vi "MapURLCreation.vi"(1 "Longitude":dbl=-1.307 format="%#.6g", 2 "Latitude":dbl=51.4062 format="%#.6g") -> (0 "URL":string="http://maps.google.com/staticmap?center=51.406200,-1.307000&zoom=18&size=570x350&maptype=hybrid&markers=51.406200,-1.307000,midpurplea&key=&path=rgb:0xFF1000,weight:5|51.406200,-1.307000|51.406200,-1.307000")   [LabVIEW 2015]
panel:
  # "Balloon Position"
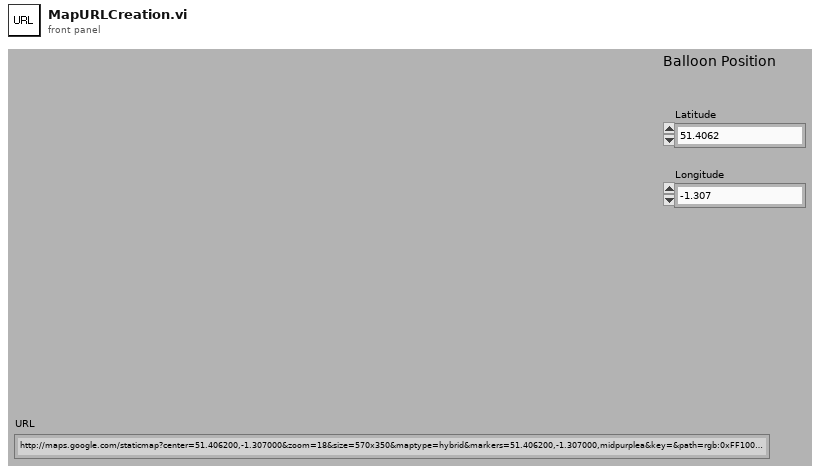
[diagram p1: front panel]
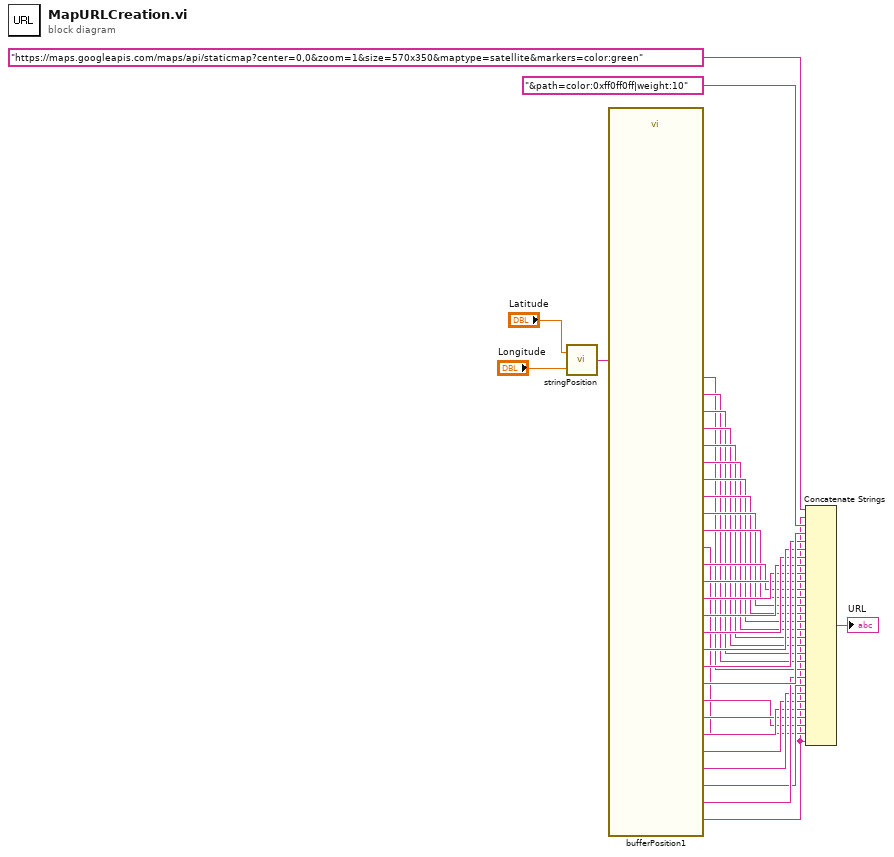
[diagram p0: block diagram]
diagram:
  n1 = call "stringPosition.vi"("Longitude"="Longitude", "Latitude"="Latitude") -> ("StringPosition"=w28:string)
  n2 = call "bufferPosition1.vi"("Input String"=w28) -> ("Output 21"=w21:string, "Output 22"=w22:string, "Output 23"=w23:string, "Output 24"=w24:string, "Output 27"=w27:string, "Output 25"=w25:string, "Output 26"=w26:string, "Output 16"=w16:string, "Output 20"=w20:string, "Output 15"=w15:string, "Output 19"=w19:string, "Output 14"=w14:string, "Output 18"=w18:string, "Output 13"=w13:string, "Output 17"=w17:string, "Output 12"=w12:string, "Output1"=w1:string, "Output 11"=w11:string, "Output 2"=w2:string, "Output 10"=w10:string, "Output 9"=w9:string, "Output 8"=w8:string, "Output 7"=w7:string, "Output 6"=w6:string, "Output 5"=w5:string, "Output 4"=w4:string, "Output 3"=w3:string)
  n3 = Concatenate Strings("https://maps.googleapis.com/maps/api/staticmap?center=0,0&zoom=1&size=570x350&maptype=satellite&markers=color:green" ("URL"), w1, "&path=color:0xff0ff0ff|weight:10", w27, w26, w25, w24, w23, w22, w21, w20, w19, w18, w17, w16, w15, w14, w13, w12, w11, w10, w9, w8, w7, w6, w5, w4, w3, w2, w1) -> (→"URL":string)
